vi "OnUpdate.vi"(8 "error in (no error)":errorcluster) -> (0 "error out":errorcluster)   [LabVIEW 2020, in "WebServiceImporter.lvlib" / "Main Panel.lvlib" / "Input WSDL.lvlib"]
uses:
  <vilib>/Platform/WebService/Main Panel/Pages/Input WSDL/Input WSDL.lvlib
  <vilib>/Platform/WebService/Main Panel/Pages/Input WSDL/Events/Events.lvlib
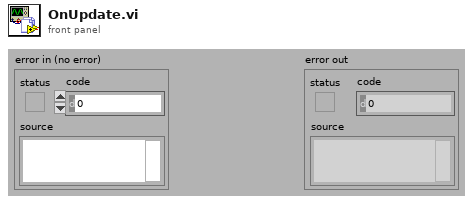
[diagram p1: front panel]
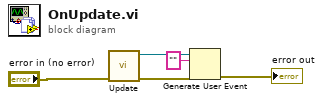
[diagram p0: block diagram]
diagram:
  n1 = call <vilib>:"Update.vi"("error in (no error)"="error in (no error)") -> ("error out"=w2:errorcluster, "user event (out)"=w3:refnum<user-event>)  [unwired: 9 in]
  n2 = Generate User Event(user event=w3, event data cluster="" ("event data"), error in=w2) -> (error out=→"error out":errorcluster)  [unwired: 1 in, 1 out]
